vi "VI Tree.vi"   [LabVIEW 2019, in "9103Series.lvlib"]
doc: "This is the instrument driver for the <INSTRUMENT NAME>. The VI Tree displays all the user-callable VIs of the instrument driver in an organized table."
uses:
  <instrlib>/9103Series/9103Series.lvlib
panel:
  # "(c) 2020 B&K Precision.  ALL RIGHTS RESERVED."
  # "SEE DIAGRAM\nFOR VI TREE."
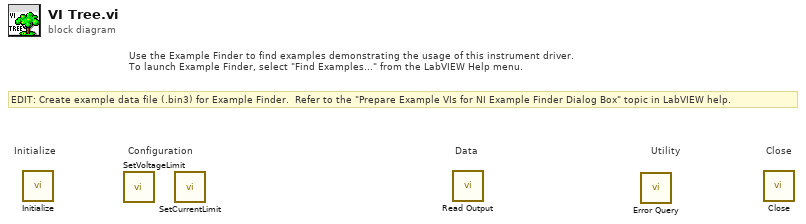
[diagram p0: block diagram]
diagram:
  # "EDIT: Create example data file (.bin3) for Example Finder.  Refer to the \"Prepare Example VIs for NI Example Finder Dialog Box\" topic in LabVIEW help."
  # "Use the Example Finder to find examples demonstrating the usage of this instrument driver.\nTo launch Example Finder, select \"Find Examples...\" from the LabVIEW Help menu."
  # "Configuration"
  # "Utility"
  # "Data"
  # "Close"
  # "Initialize"
  n1 = call <instrlib>:"Initialize.vi"() -> ()  [unwired: 10 in, 2 out]
  n2 = call <instrlib>:"SetVoltageLimit.vi"() -> ()  [unwired: 12 in]
  n3 = call <instrlib>:"SetCurrentLimit.vi"() -> ()  [unwired: 12 in]
  n4 = call <instrlib>:"Read Output.vi"() -> ()  [unwired: 12 in]
  n5 = call <instrlib>:"Error Query.vi"() -> ()  [unwired: 8 in, 4 out]
  n6 = call <instrlib>:"Close.vi"() -> ()  [unwired: 11 in, 1 out]
